vi "Command Picture.vi"(5 "Unused":bool, 7 "Feedback State":T1, 10 "Command State":T1, 11 "Command Pictures":T3) -> (2 "Command Picture":T2)   [LabVIEW 2020, in "VolatusGUIElements.lvlib" / "2WayValveH.lvclass"]
uses:
  2WayValveH.lvclass
  Channel State.ctl
  Command Pictures.ctl
  Picture.ctl
  2WayValveH.lvclass/2WayValveH.ctl
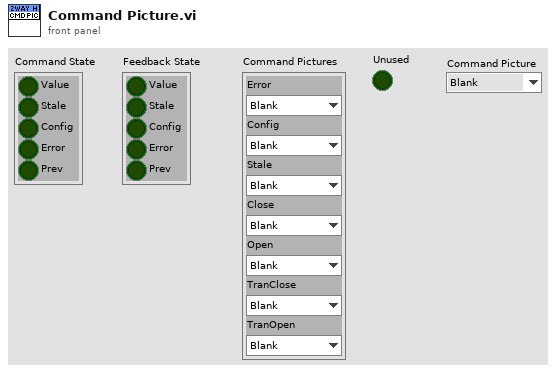
[diagram p1: front panel]
types:
  T1 = typedef "VolatusGUIElements.lvlib/2WayValveH.lvclass/Channel State.ctl" = cluster{"Value":bool, "Stale":bool, "Config":bool, "Error":bool, "Prev":bool}
  T2 = typedef "VolatusGUIElements.lvlib/2WayValveH.lvclass/Picture.ctl" = enum16{"Blank", "OutClose", "OutOpen", "OutTranClose", "OutTranOpen", "OutConfig", "OutStale", "OutError", "InClose", "InOpen", "InTranClose", "InTranOpen", "InConfig", "InStale", "InError", "EnOff", "EnOn", "EnConfig", "EnStale", "EnError"}
  T3 = typedef "VolatusGUIElements.lvlib/2WayValveH.lvclass/Command Pictures.ctl" = cluster{"Error":T2, "Config":T2, "Stale":T2, "Close":T2, "Open":T2, "TranClose":T2, "TranOpen":T2}
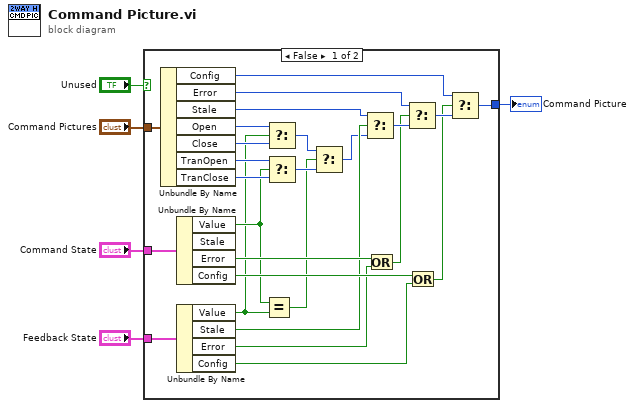
[diagram p0: block diagram]
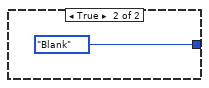
[diagram p2: hidden frame]
diagram:
  n1 = case shown="False" "Unused" {
    tunnel: "Command State" -> [w31 _]
    tunnel: "Command Pictures" -> [w30 _]
    tunnel: [w22 Picture."Blank" ("Close")] -> w3
    tunnel: "Feedback State" -> [w17 _]
    frame False {
      n2 = Unbundle By Name(w30) -> ("Config"=w23:T2, "Error"=w24:T2, "Stale"=w27:T2, "Open"=w28:T2, "Close"=w29:T2, "TranOpen"=w13:T2, "TranClose"=w12:T2)
      n3 = Unbundle By Name(w31) -> ("Value"=w11:bool, "Error"=w21:bool, "Config"=w19:bool)  [unwired: 1 out]
      n4 = Unbundle By Name(w17) -> ("Value"=w10:bool, "Stale"=w16:bool, "Error"=w15:bool, "Config"=w14:bool)
      n5 = Equal?(x=w11, y=w10) -> (x = y?=w7:bool)
      n6 = Select(t=w28, s=w10, f=w29) -> (s? t:f=w9:T2)
      n7 = Select(t=w13, s=w11, f=w12) -> (s? t:f=w8:T2)
      n8 = Select(t=w9, s=w7, f=w8) -> (s? t:f=w6:T2)
      n9 = Select(t=w27, s=w16, f=w6) -> (s? t:f=w26:T2)
      n10 = Or(x=w21, y=w15) -> (x .or. y?=w20:bool)
      n11 = Select(t=w24, s=w20, f=w26) -> (s? t:f=w25:T2)
      n12 = Or(x=w19, y=w14) -> (x .or. y?=w18:bool)
      n13 = Select(t=w23, s=w18, f=w25) -> (s? t:f=w22:T2)
    }
    frame True {
    }
  }
  "Command Picture" <- w3
